vi "Get Voltage.vi"(8 "error in":errorcluster, 11 "DAQ HVPS in":refnum<class "DAQ HVPS.lvclass">) -> (0 "error out":errorcluster, 2 "V":dbl, 3 "DAQ HVPS out":refnum<class "DAQ HVPS.lvclass">)   [LabVIEW 2014, in "DAQ HVPS.lvclass"]
doc: "Retrieve a finite number of samples from the DAQ device, average those samples and return a voltage."
uses:
  DAQ HVPS.lvclass
  DAQ HVPS.lvclass/DAQ HVPS.ctl
  <vilib>/Analysis/baseanly.llb/Mean (DBL).vi
  <vilib>/DAQmx/read.llb/DAQmx Read (Analog 1D DBL 1Chan NSamp).vi
  <vilib>/Analysis/NI_AALBase.lvlib
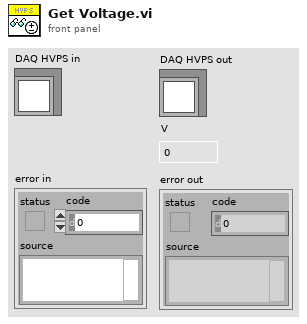
[diagram p1: front panel]
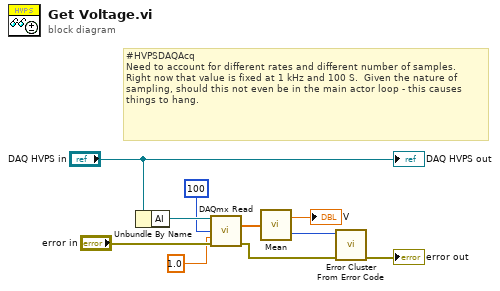
[diagram p0: block diagram]
diagram:
  # "#HVPSDAQAcq\nNeed to account for different rates and different number of samples.  Right now that value is fixed at 1 kHz and 100 S.  Given the nature of sampling, should this not even be in the main actor loop - this causes things to hang."
  n1 = Unbundle By Name("DAQ HVPS in") -> ("AI"=w7:refnum<k21>)
  n2 = call-poly <vilib>:"DAQmx Read.vi"("task/channels in"=w7, "number of samples per channel"=100, "timeout"=1.0, "error in"="error in") -> ("data"=w4:dbl[], "error out"=w1:errorcluster)  [unwired: 9 in, 1 out]
  n3 = call-poly <vilib>:"Mean.vi"("X"=w4) -> ("mean"=→"V":dbl, "error"=w2:i32)
  n4 = call <vilib>:"Error Cluster From Error Code.vi"("error in (no error)"=w1, "error code (0)"=w2) -> ("error out"=→"error out":errorcluster)  [unwired: 7 in]
  "DAQ HVPS out" <- "DAQ HVPS in"
